vi "myRIO_BRig_RT_dataLC_Cue1_OnOff_NS_l2.vi"() -> (2 "output_Cue1_OnOff_NS_l2":i32)   [LabVIEW 2014]
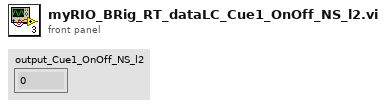
[diagram p1: front panel]
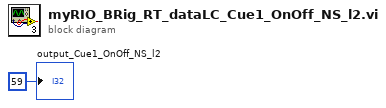
[diagram p0: block diagram]
diagram:
  "output_Cue1_OnOff_NS_l2" <- 59 ("output_iBlock")
